vi "restore_config.vi"   [LabVIEW 2011]
doc: "Restores the chirp pulse experiment settings from a config file."
uses:
  <vilib>/Utility/config.llb/Read Key (I32).vi
  global.vi
  <vilib>/Utility/config.llb/Read Key (Boolean).vi
  <vilib>/Utility/config.llb/Read Key (Double).vi
  <vilib>/Utility/config.llb/Read Key (String).vi
  <vilib>/Utility/config.llb/NI_LVConfig.lvlib
types:
  T1 = typedef "NI_LVConfig.lvlib/Config Data RefNum.ctl" = refnum<k1>
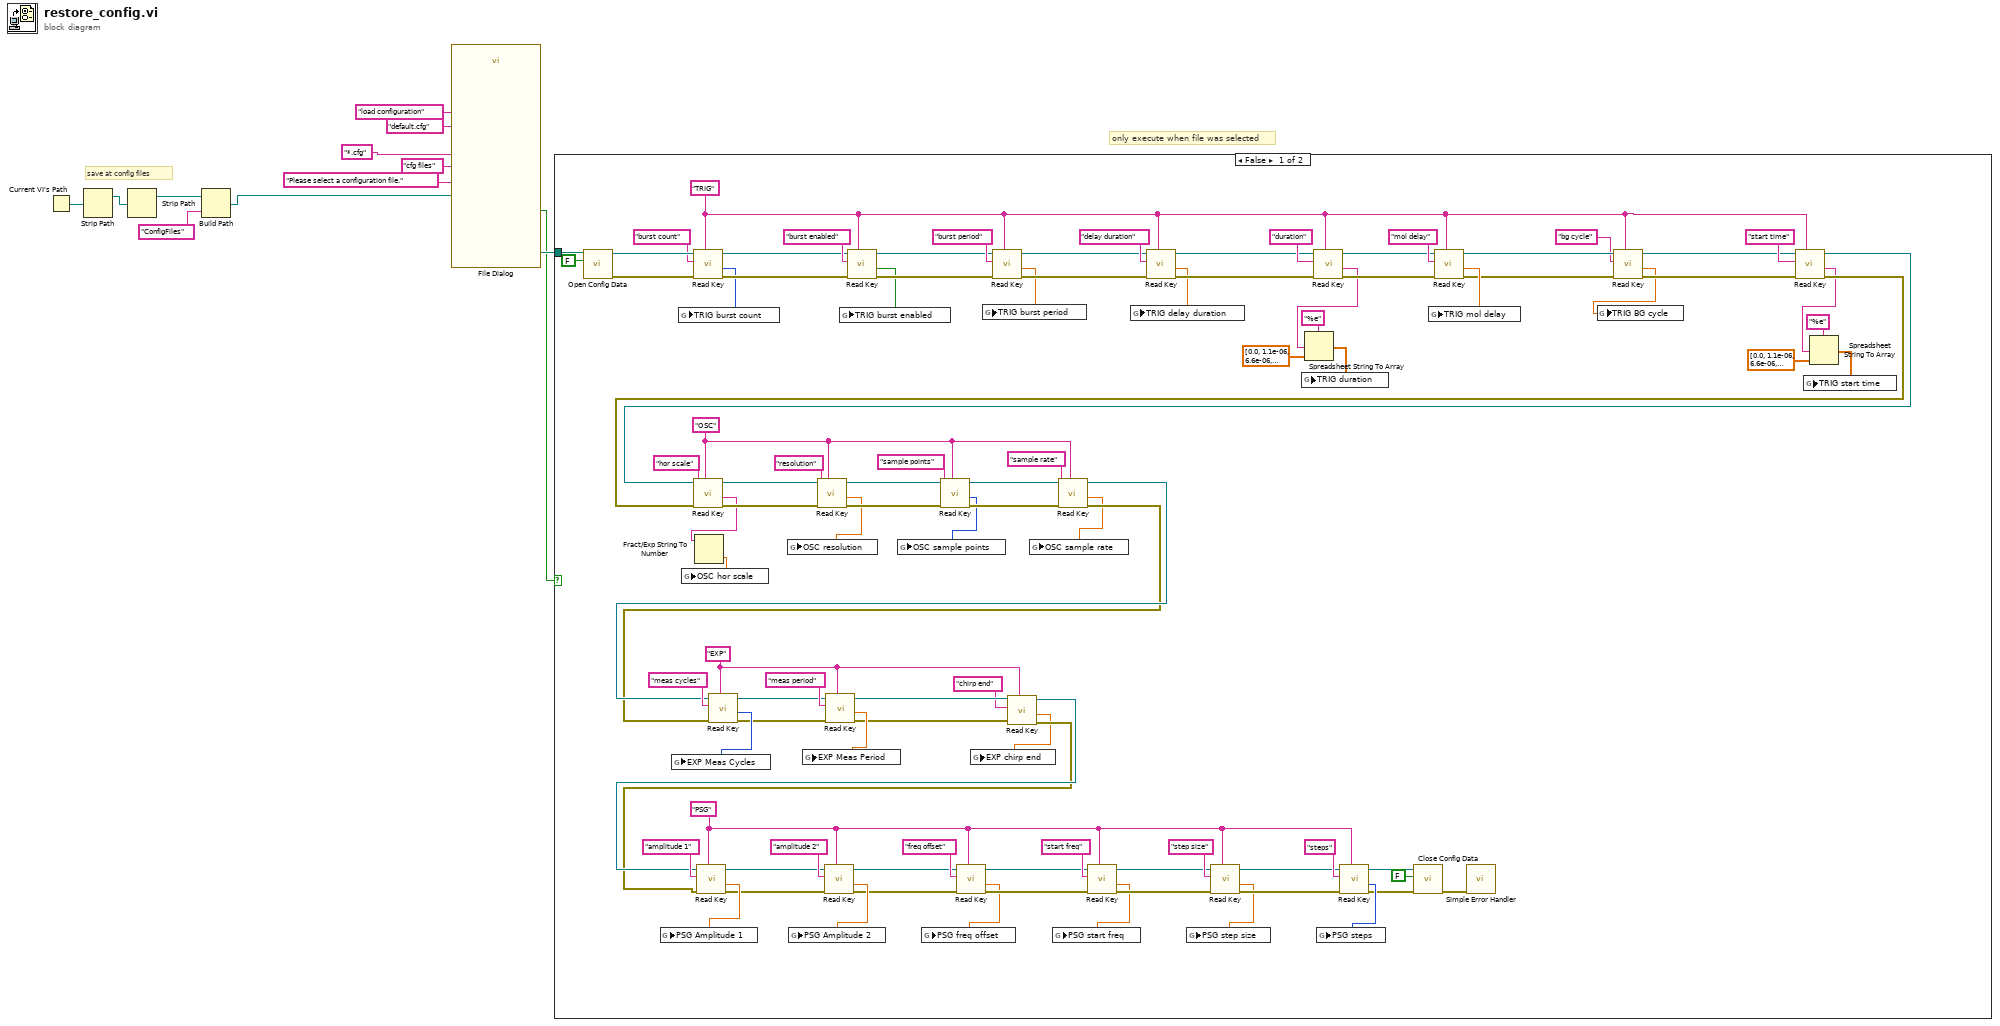
[diagram p0: block diagram]
diagram:
  # "only execute when file was selected"
  # "save at config files"
  n1 = Current VI's Path() -> (path=w6:path)
  n2 = Strip Path(path=w6) -> (stripped path=w4:path)  [unwired: 1 out]
  n3 = Strip Path(path=w4) -> (stripped path=w3:path)  [unwired: 1 out]
  n4 = Build Path(base path=w3, name or relative path="ConfigFiles") -> (appended path=w2:path)
  n5 = call "File Dialog"("start path"=w2, "prompt"="Please select a configuration file.", "button label"="load configuration", "default name"="default.cfg", "pattern (all files)"="*.cfg" ("default name"), "pattern label"="cfg files") -> ("selected path"=w12:path, "cancelled"=w1:bool)  [unwired: 6 in, 2 out]
  n6 = case shown="False" w1 {
    tunnel: w12 -> [w109 _]
    frame False {
      w39 = "PSG"
      w15 = "EXP"
      w80 = "OSC"
      w26 = "TRIG"
      n7 = call <vilib>:"Open Config Data.vi"("create file if necessary (T)"=FALSE, "configuration file path"=w109) -> ("error out"=w112:errorcluster, "refnum"=w113:T1)  [unwired: 1 in, 7 out]
      n8 = call-poly <vilib>:"Read Key.vi"("section"=w26, "error in (no error)"=w112, "key"="burst count" ("Key 1"), "refnum"=w113) -> ("error out"=w100:errorcluster, "value"=w65:i32, "refnum out"=w104:T1)  [unwired: 4 in, 1 out]
      n9 = global write "global.vi" "TRIG burst count"(w65) -> ()
      n10 = call-poly <vilib>:"Read Key.vi"("section"=w26, "error in (no error)"=w100, "key"="burst enabled" ("Key 1"), "refnum"=w104) -> ("error out"=w99:errorcluster, "value"=w64:bool, "refnum out"=w103:T1)  [unwired: 4 in, 1 out]
      n11 = global write "global.vi" "TRIG burst enabled"(w64) -> ()
      n12 = call-poly <vilib>:"Read Key.vi"("section"=w26, "error in (no error)"=w99, "key"="burst period" ("Key 1"), "refnum"=w103) -> ("error out"=w98:errorcluster, "value"=w63:dbl, "refnum out"=w102:T1)  [unwired: 4 in, 1 out]
      n13 = global write "global.vi" "TRIG burst period"(w63) -> ()
      n14 = call-poly <vilib>:"Read Key.vi"("section"=w26, "error in (no error)"=w98, "key"="delay duration" ("Key 1"), "refnum"=w102) -> ("error out"=w97:errorcluster, "value"=w62:dbl, "refnum out"=w101:T1)  [unwired: 4 in, 1 out]
      n15 = global write "global.vi" "TRIG delay duration"(w62) -> ()
      n16 = call-poly <vilib>:"Read Key.vi"("section"=w26, "error in (no error)"=w97, "key"="duration" ("Key 1"), "refnum"=w101) -> ("error out"=w93:errorcluster, "value"=w59:string, "refnum out"=w94:T1)  [unwired: 4 in, 1 out]
      n17 = Spreadsheet String To Array(format string="%e", spreadsheet string=w59, array type (2D Dbl)=dbl[] [0.0, 1.1e-06, 6.6e-06, 6.4e-06] ("TRIG start time")) -> (array=w60:dbl[])  [unwired: 1 in]
      n18 = global write "global.vi" "TRIG duration"(w60) -> ()
      n19 = call-poly <vilib>:"Read Key.vi"("section"=w26, "error in (no error)"=w93, "key"="mol delay" ("Key 1"), "refnum"=w94) -> ("error out"=w23:errorcluster, "value"=w54:dbl, "refnum out"=w22:T1)  [unwired: 4 in, 1 out]
      n20 = global write "global.vi" "TRIG mol delay"(w54) -> ()
      n21 = call-poly <vilib>:"Read Key.vi"("section"=w26, "error in (no error)"=w23, "key"="bg cycle" ("Key 1"), "refnum"=w22) -> ("error out"=w24:errorcluster, "value"=w20:dbl, "refnum out"=w25:T1)  [unwired: 4 in, 1 out]
      n22 = global write "global.vi" "TRIG BG cycle"(w20) -> ()
      n23 = call-poly <vilib>:"Read Key.vi"("section"=w26, "error in (no error)"=w24, "key"="start time" ("Key 1"), "refnum"=w25) -> ("error out"=w85:errorcluster, "value"=w53:string, "refnum out"=w84:T1)  [unwired: 4 in, 1 out]
      n24 = call-poly <vilib>:"Read Key.vi"("section"=w80, "error in (no error)"=w85, "key"="hor scale" ("Key 1"), "refnum"=w84) -> ("error out"=w87:errorcluster, "value"=w32:string, "refnum out"=w89:T1)  [unwired: 4 in, 1 out]
      n25 = Fract/Exp String To Number(string=w32) -> (number=w31:dbl)  [unwired: 3 in, 1 out]
      n26 = global write "global.vi" "OSC hor scale"(w31) -> ()
      n27 = call-poly <vilib>:"Read Key.vi"("section"=w80, "error in (no error)"=w87, "key"="resolution" ("Key 1"), "refnum"=w89) -> ("error out"=w86:errorcluster, "value"=w52:dbl, "refnum out"=w88:T1)  [unwired: 4 in, 1 out]
      n28 = global write "global.vi" "OSC resolution"(w52) -> ()
      n29 = call-poly <vilib>:"Read Key.vi"("section"=w80, "error in (no error)"=w86, "key"="sample points" ("Key 1"), "refnum"=w88) -> ("error out"=w81:errorcluster, "value"=w51:i32, "refnum out"=w82:T1)  [unwired: 4 in, 1 out]
      n30 = global write "global.vi" "OSC sample points"(w51) -> ()
      n31 = call-poly <vilib>:"Read Key.vi"("section"=w80, "error in (no error)"=w81, "key"="sample rate" ("Key 1"), "refnum"=w82) -> ("error out"=w77:errorcluster, "value"=w50:dbl, "refnum out"=w78:T1)  [unwired: 4 in, 1 out]
      n32 = call-poly <vilib>:"Read Key.vi"("section"=w15, "error in (no error)"=w77, "key"="meas cycles" ("Key 1"), "refnum"=w78) -> ("error out"=w28:errorcluster, "value"=w49:i32, "refnum out"=w29:T1)  [unwired: 4 in, 1 out]
      n33 = global write "global.vi" "EXP Meas Cycles"(w49) -> ()
      n34 = call-poly <vilib>:"Read Key.vi"("section"=w15, "error in (no error)"=w28, "key"="meas period" ("Key 1"), "refnum"=w29) -> ("error out"=w17:errorcluster, "value"=w27:dbl, "refnum out"=w16:T1)  [unwired: 4 in, 1 out]
      n35 = global write "global.vi" "EXP Meas Period"(w27) -> ()
      n36 = call-poly <vilib>:"Read Key.vi"("section"=w15, "error in (no error)"=w17, "key"="chirp end", "refnum"=w16) -> ("error out"=w18:errorcluster, "value"=w14:dbl, "refnum out"=w19:T1)  [unwired: 4 in, 1 out]
      n37 = call-poly <vilib>:"Read Key.vi"("section"=w39, "error in (no error)"=w18, "key"="amplitude 1" ("Key 1"), "refnum"=w19) -> ("error out"=w34:errorcluster, "value"=w42:dbl, "refnum out"=w36:T1)  [unwired: 4 in, 1 out]
      n38 = global write "global.vi" "PSG Amplitude 1"(w42) -> ()
      n39 = call-poly <vilib>:"Read Key.vi"("section"=w39, "error in (no error)"=w34, "key"="amplitude 2" ("Key 1"), "refnum"=w36) -> ("error out"=w33:errorcluster, "value"=w40:dbl, "refnum out"=w35:T1)  [unwired: 4 in, 1 out]
      n40 = global write "global.vi" "PSG Amplitude 2"(w40) -> ()
      n41 = call-poly <vilib>:"Read Key.vi"("section"=w39, "error in (no error)"=w33, "key"="freq offset" ("Key 1"), "refnum"=w35) -> ("error out"=w71:errorcluster, "value"=w48:dbl, "refnum out"=w73:T1)  [unwired: 4 in, 1 out]
      n42 = global write "global.vi" "PSG freq offset"(w48) -> ()
      n43 = global write "global.vi" "EXP chirp end"(w14) -> ()
      n44 = global write "global.vi" "OSC sample rate"(w50) -> ()
      n45 = call-poly <vilib>:"Read Key.vi"("section"=w39, "error in (no error)"=w71, "key"="start freq" ("Key 1"), "refnum"=w73) -> ("error out"=w70:errorcluster, "value"=w47:dbl, "refnum out"=w72:T1)  [unwired: 4 in, 1 out]
      n46 = global write "global.vi" "PSG start freq"(w47) -> ()
      n47 = call-poly <vilib>:"Read Key.vi"("section"=w39, "error in (no error)"=w70, "key"="step size" ("Key 1"), "refnum"=w72) -> ("error out"=w67:errorcluster, "value"=w46:dbl, "refnum out"=w68:T1)  [unwired: 4 in, 1 out]
      n48 = global write "global.vi" "PSG step size"(w46) -> ()
      n49 = call-poly <vilib>:"Read Key.vi"("section"=w39, "error in (no error)"=w67, "key"="steps" ("Key 1"), "refnum"=w68) -> ("error out"=w37:errorcluster, "value"=w45:i32, "refnum out"=w38:T1)  [unwired: 4 in, 1 out]
      n50 = global write "global.vi" "PSG steps"(w45) -> ()
      n51 = call <vilib>:"Close Config Data.vi"("error in (no error)"=w37, "write file if changed (T)"=FALSE, "refnum"=w38) -> ("error out"=w110:errorcluster)  [unwired: 8 out]
      n52 = call <vilib>:"Simple Error Handler.vi"("error in (no error)"=w110) -> ()  [unwired: 1 in, 8 out]
      n53 = Spreadsheet String To Array(format string="%e", spreadsheet string=w53, array type (2D Dbl)=dbl[] [0.0, 1.1e-06, 6.6e-06, 6.4e-06] ("TRIG start time")) -> (array=w56:dbl[])  [unwired: 1 in]
      n54 = global write "global.vi" "TRIG start time"(w56) -> ()
    }
    frame True {
    }
  }
